vi "MP alias.vi"(11 "Philosopher in":refnum<class "Philosopher.lvclass">) -> (3 "MP Alias":string)   [LabVIEW 2021, in "Philosopher.lvclass"]
uses:
  Philosopher.lvclass
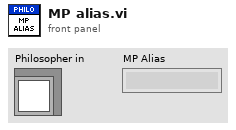
[diagram p1: front panel]
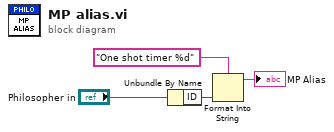
[diagram p0: block diagram]
diagram:
  n1 = Unbundle By Name("Philosopher in") -> ("ID"=w2:i32)
  n2 = Format Into String(format string="One shot timer %d" ("Worker Alias"), w2) -> (resulting string=→"MP Alias":string)  [unwired: 2 in, 1 out]
